vi "UART Number.vi"(4 "UART in":refnum<class "UART.lvclass">) -> (7 "UART #":T1=-1)   [LabVIEW 2024, in "CTI.lvlib" / "UART.lvclass"]
uses:
  UART.lvclass
  UART Number.ctl
  UART.lvclass/UART.ctl
  CTI.lvlib
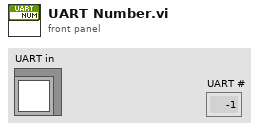
[diagram p1: front panel]
types:
  T1 = typedef "CTI.lvlib/UART Number.ctl" = i8
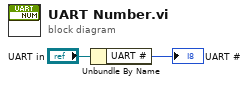
[diagram p0: block diagram]
diagram:
  n1 = Unbundle By Name("UART in") -> ("UART #"=→"UART #":T1)
